vi "未命名 1.vi"() -> ()   [LabVIEW 2013]
panel:
  out "error out":errorcluster
  out "区域最大位移1(mm)":dbl format="%#.1f"
  out "区域最小位移1(mm)":dbl format="%#.1f"
  out "区域最大压力1(KN)":dbl format="%#.3f"
  out "位移监控点1(mm)":dbl format="%#.1f"
  out "监控点最小压力1(KN)":dbl format="%#.3f"
  out "监控点最大压力1(KN)":dbl format="%#.3f"
  out "最小压入位移1(mm)":dbl format="%#.1f"
  out "最大压入位移1(mm)":dbl format="%#.1f"
  out "区域最小压力1(KN)":dbl format="%#.3f"
  out "区域最小压力2(KN)":dbl format="%#.3f"
  out "最小压入位移2(mm)":dbl format="%#.1f"
  out "最大压入位移2(mm)":dbl format="%#.1f"
  out "区域最大压力2(KN)":dbl format="%#.3f"
  out "位移监控点2(mm)":dbl format="%#.1f"
  out "监控点最大压力2(KN)":dbl format="%#.3f"
  out "监控点最小压力2(KN)":dbl format="%#.3f"
  out "区域最小位移2(mm)":dbl format="%#.1f"
  out "区域最大位移2(mm)":dbl format="%#.1f"
  out "伺服1位置设置":dbl format="%#.1f"
  out "伺服2位置设置":dbl format="%#.1f"
  out "吹气时间设置":dbl
  out "喷油时间设置":dbl
  out "伺服2速度设置":dbl format="%#.1f"
  out "伺服1速度设置":dbl format="%#.1f"
  in  "参数加载":bool
  out "ADODB._Connection Out":refnum<k7>
  in  "位移2零点偏移值":dbl format="%#.3f"
  in  "位移2比例偏移值":dbl format="%#.3f"
  in  "压力2比例偏移值":dbl format="%#.3f"
  in  "压力2零点偏移值":dbl format="%#.3f"
  in  "位移1零点偏移值":dbl format="%#.3f"
  in  "位移1比例偏移值":dbl format="%#.3f"
  in  "压力1比例偏移值":dbl format="%#.3f"
  in  "压力1零点偏移值":dbl format="%#.3f"
  in  "停止":bool
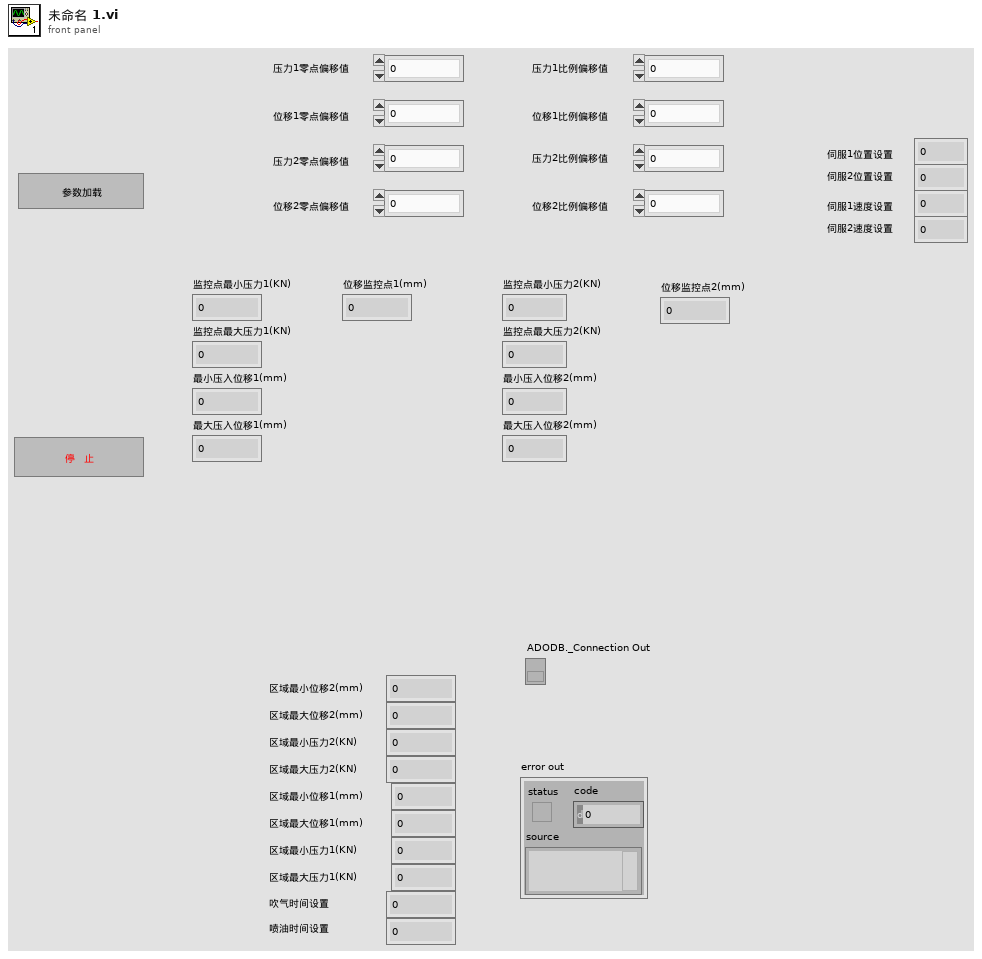
[diagram p1: front panel]
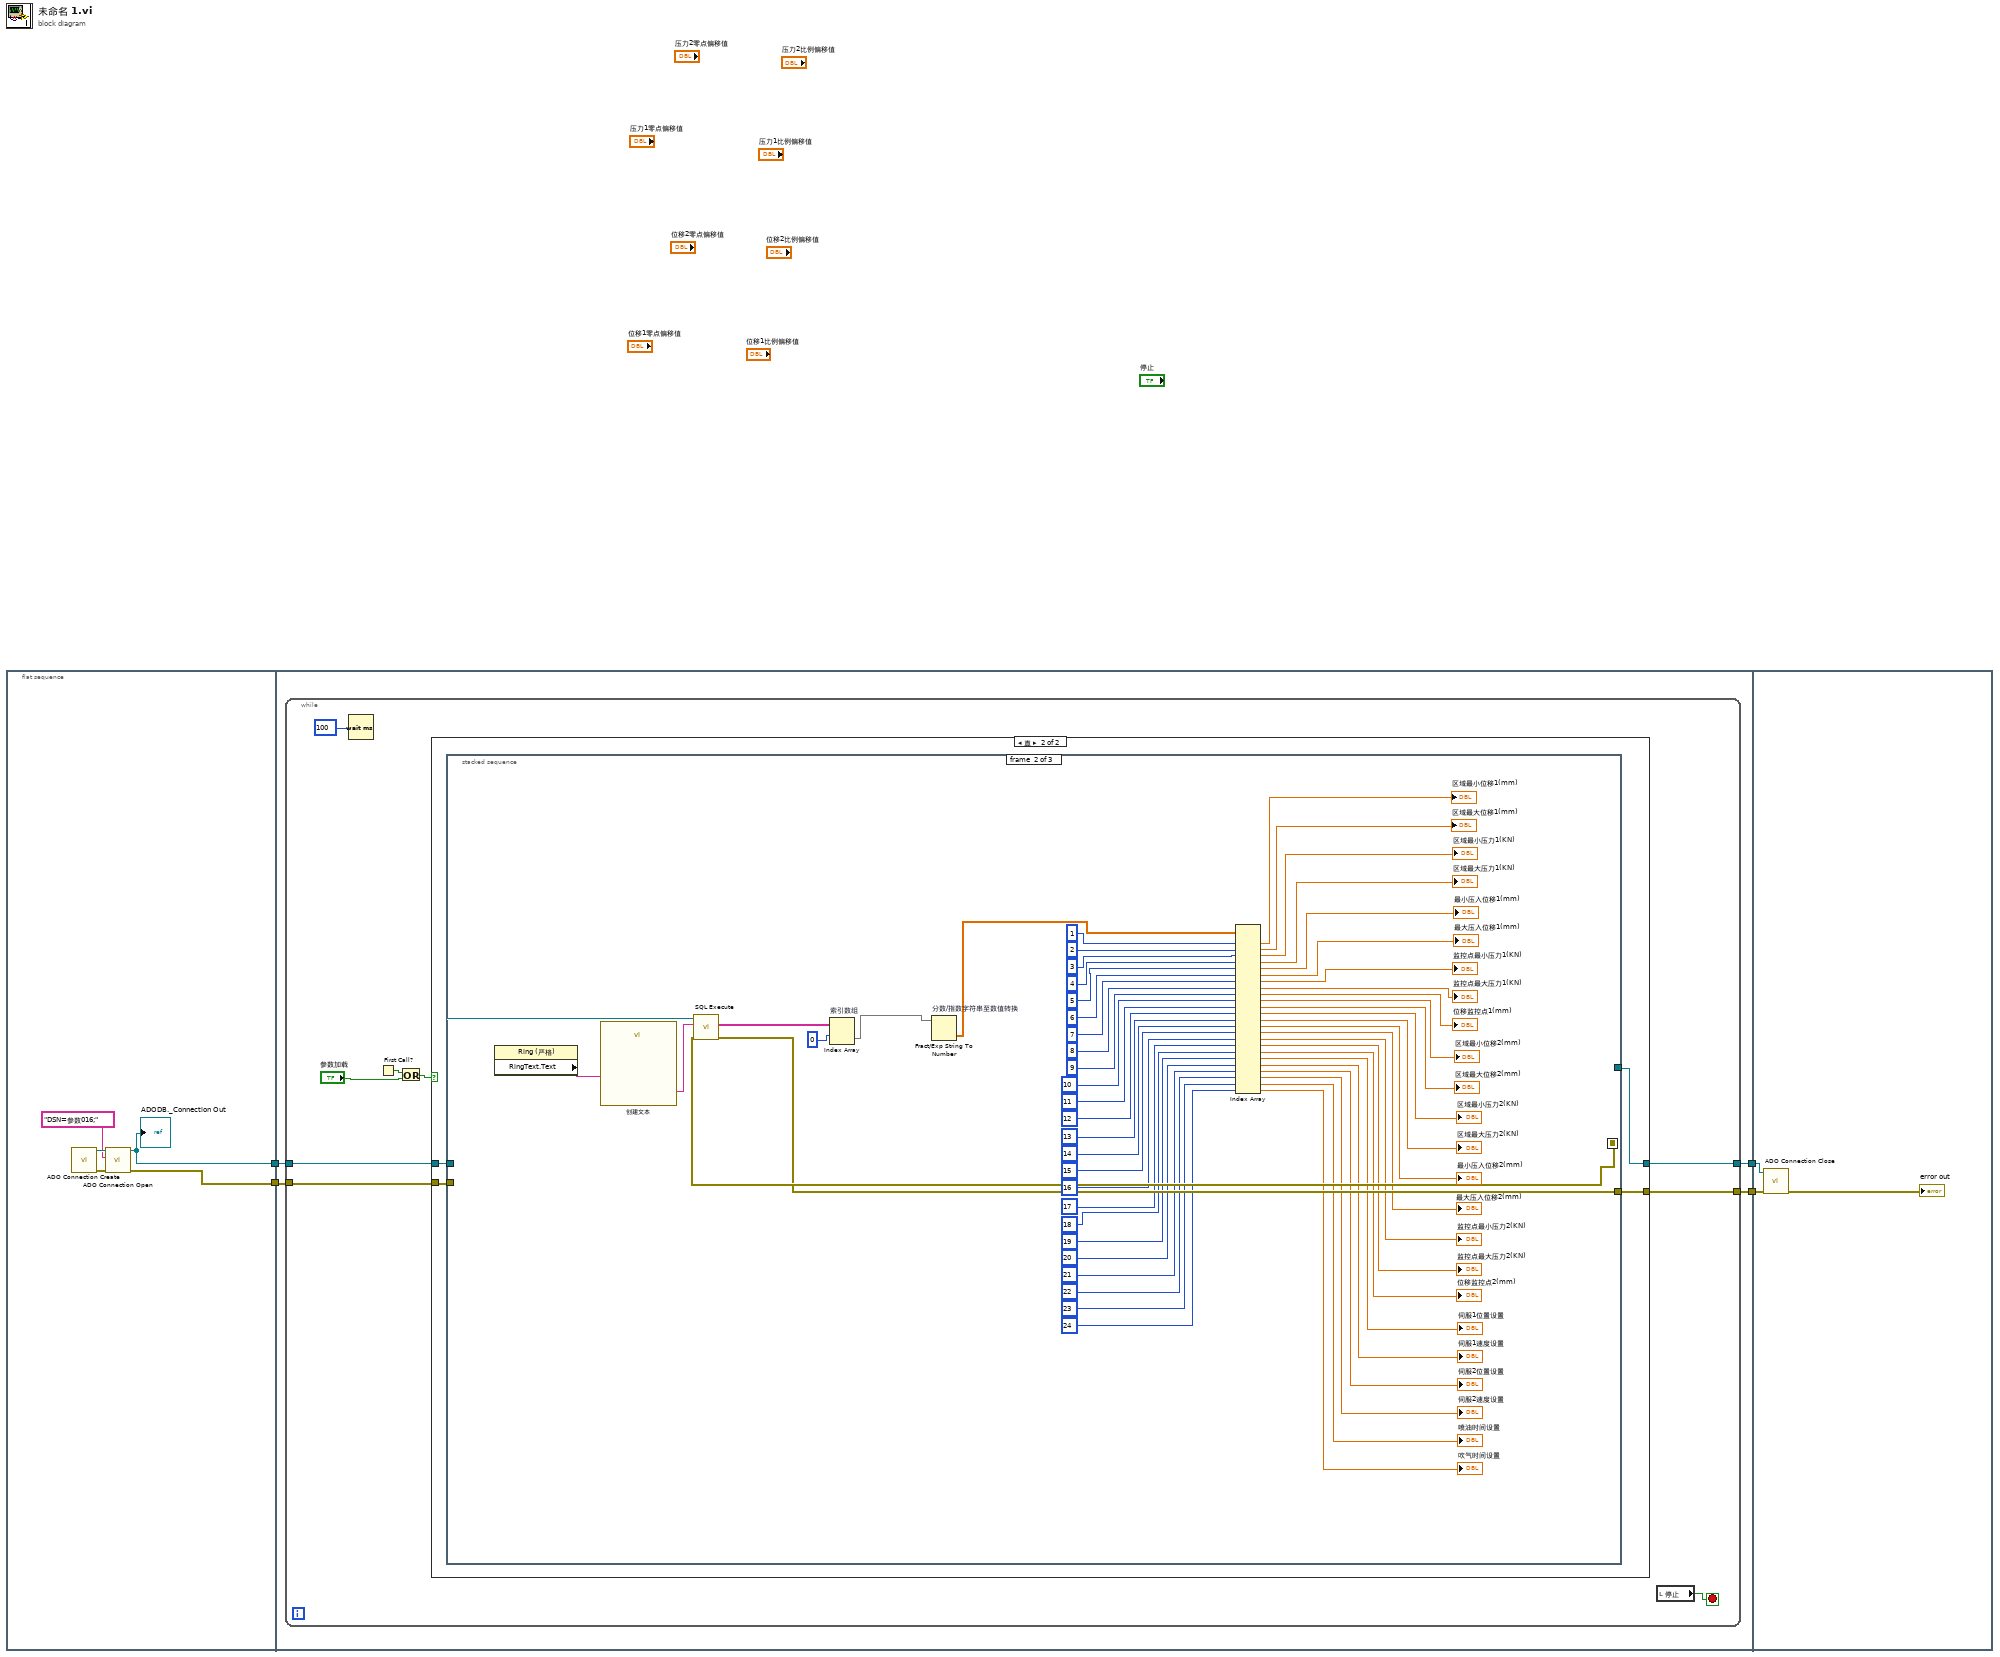
[diagram p0: block diagram]
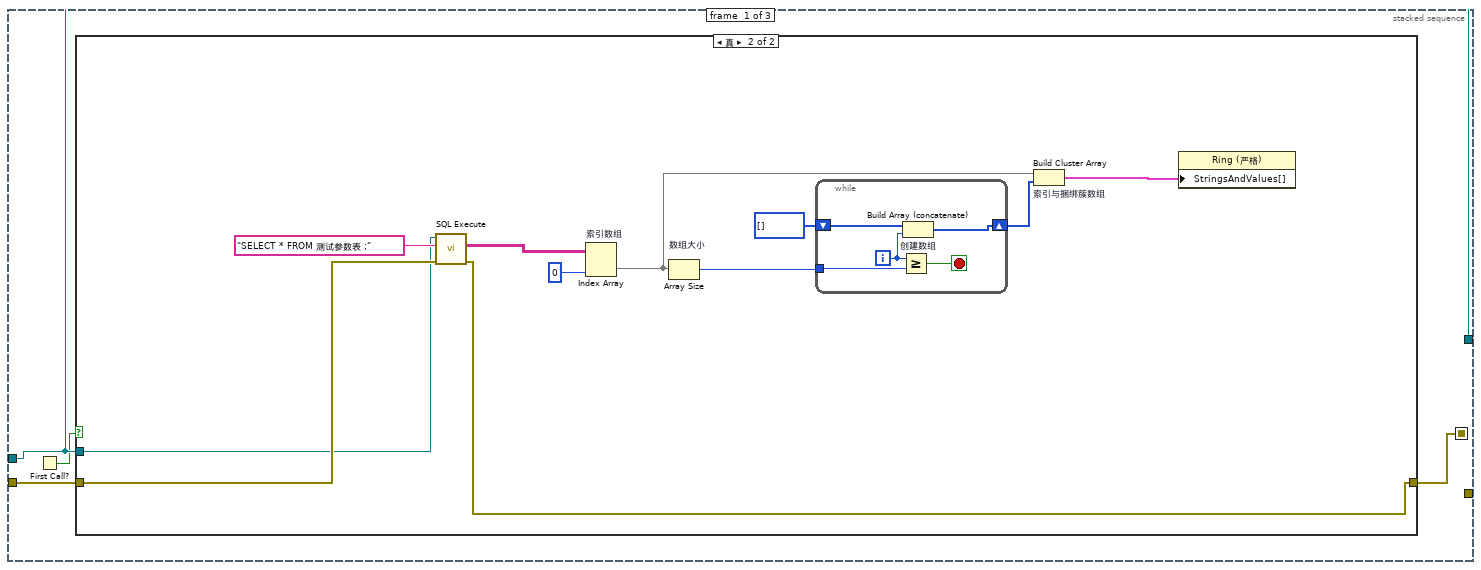
[diagram p3: hidden frame]
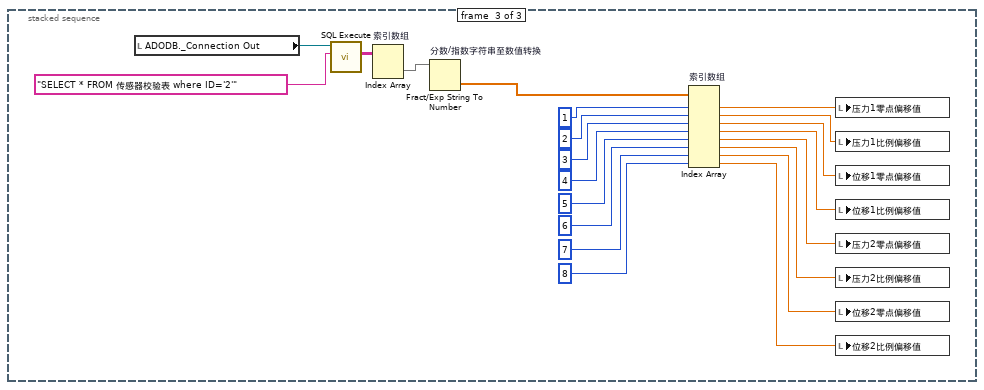
[diagram p5: hidden frame]
diagram:
  n1 = flat-sequence {
    tunnel: [w6] -> w4
    tunnel: [w5] -> w3
    tunnel: w4 -> [w13]
    tunnel: w3 -> [w12]
    tunnel: [w11] -> w2
    tunnel: [w10] -> w1
    tunnel: w2 -> [w129]
    tunnel: w1 -> [w128]
    frame #0 {
      n2 = call "ADO Connection Create.vi"() -> ("error out"=w8:errorcluster, "ADODB._Connection Out"=w9:refnum<k7>)  [unwired: 10 in]
      n3 = call "ADO Connection Open.vi"("error in (no error)"=w8, "ConnectionString"="DSN=参数016;", "ADODB._Connection In"=w9) -> ("error out"=w5:errorcluster, "ADODB._Connection Out"=w6:refnum<k7>)  [unwired: 7 in]
      "ADODB._Connection Out" <- w6
    }
    frame #1 {
      n4 = while {
        tunnel: w13 -> [w18]
        tunnel: w12 -> [w17]
        tunnel: [w16] -> w11
        tunnel: [w15] -> w10
        stop <- w21 stop-if-true
        n5 = Wait (ms)(milliseconds to wait=u32 100 ("等待时间（毫秒）")) -> ()  [unwired: 1 out]
        n6 = First Call?() -> (First Call?: T/F=w20:bool)
        n7 = Or(x=w20, y="参数加载") -> (x .or. y?=w19:bool)
        n8 = case shown="真" w19 {
          tunnel: w18 -> [w24 w28]
          tunnel: w17 -> [w23 w27]
          tunnel: [w24 w26] -> w16
          tunnel: [w23 w25] -> w15
          frame False {
          }
          frame True {
            n9 = stacked-sequence {
              seq-local: [w29 _ _] -> [_ w104 _]
              tunnel: w28 -> [w31 w101 _]
              tunnel: w27 -> [w32 _ _]
              tunnel: [w31 _ _] -> w26
              tunnel: [_ w103 _] -> w25
              frame #0 {
                n10 = First Call?() -> (First Call?: T/F=w30:bool)
                n11 = case shown="真" w30 {
                  tunnel: w32 -> [w33 w38]
                  tunnel: w31 -> [_ w36]
                  tunnel: [w33 w35] -> w29
                  frame False {
                  }
                  frame True {
                    n12 = call "SQL Execute.vi"("error in (no error)"=w38, "Command Text"="SELECT * FROM 测试参数表 ;", "ADODB._Connection In"=w36) -> ("error out"=w35:errorcluster, "Data"=w39:string[][])  [unwired: 5 in, 2 out]
                    n13 = Index Array "索引数组"(array=w39, index (col)=0 ("禁用的索引 (列)")) -> (element=w42:string[])  [unwired: 1 in]
                    n14 = Array Size "数组大小"(array=w42) -> (size(s)=w41:i32)
                    n15 = while {
                      shift-right: [w47] -> w40
                      shift-left: i32[] [] -> [w48]
                      tunnel: w41 -> [w45]
                      i -> [w46]
                      stop <- w49 stop-if-true
                      n16 = Greater Or Equal?(x=w46, y=w45) -> (x >= y?=w49:bool)
                      n17 = Build Array (concatenate) "创建数组"(w48, w46) -> (w47:i32[])
                    }
                    n18 = Build Cluster Array "索引与捆绑簇数组"(w42, w40) -> (w34:cluster{"String":string, i32}[])
                    n19 = property on="属性节点" class="Ring (严格)"("StringsAndValues[]"=w34) -> ()  [unwired: 2 in, 2 out]
                  }
                }
              }
              frame #1 {
                n20 = property on="属性节点" class="Ring (严格)"() -> ("RingText.Text"=w100:string)  [unwired: 2 in, 2 out]
                n21 = call "创建文本"("产品型号"=w100) -> ("Result"=w102:string)  [unwired: 13 in, 1 out]
                n22 = call "SQL Execute.vi"("error in (no error)"=w104, "Command Text"=w102, "ADODB._Connection In"=w101) -> ("error out"=w103:errorcluster, "Data"=w106:string[][])  [unwired: 5 in, 2 out]
                n23 = Index Array "索引数组"(array=w106, index (row)=0 ("索引 (行)")) -> (element=w99:string[])  [unwired: 1 in]
                n24 = Fract/Exp String To Number "分数/指数字符串至数值转换"(string=w99) -> (number=w50:dbl[])  [unwired: 3 in, 1 out]
                n25 = Index Array(array=w50, index #1=1 ("索引"), index #2=2 ("索引"), index #3=3 ("索引"), index #4=4 ("索引"), index #5=5 ("索引"), index #6=6 ("索引"), index #7=7 ("索引"), index #8=8 ("索引"), index #9=9 ("索引"), index #10=10 ("索引"), index #11=11 ("索引"), index #12=12 ("索引"), index #13=13 ("索引"), index #14=14 ("索引"), index #15=15 ("索引"), index #16=16 ("索引"), index #17=17 ("索引"), index #18=18 ("索引"), index #19=19 ("索引"), index #20=20 ("索引"), index #21=21 ("索引"), index #22=22 ("索引"), index #23=23 ("索引"), index #24=24 ("索引")) -> (element #1=→"区域最小位移1(mm)":dbl, element #2=→"区域最大位移1(mm)":dbl, element #3=→"区域最小压力1(KN)":dbl, element #4=→"区域最大压力1(KN)":dbl, element #5=→"最小压入位移1(mm)":dbl, element #6=→"最大压入位移1(mm)":dbl, element #7=→"监控点最小压力1(KN)":dbl, element #8=→"监控点最大压力1(KN)":dbl, element #9=→"位移监控点1(mm)":dbl, element #10=→"区域最小位移2(mm)":dbl, element #11=→"区域最大位移2(mm)":dbl, element #12=→"区域最小压力2(KN)":dbl, element #13=→"区域最大压力2(KN)":dbl, element #14=→"最小压入位移2(mm)":dbl, element #15=→"最大压入位移2(mm)":dbl, element #16=→"监控点最小压力2(KN)":dbl, element #17=→"监控点最大压力2(KN)":dbl, element #18=→"位移监控点2(mm)":dbl, element #19=→"伺服1位置设置":dbl, element #20=→"伺服1速度设置":dbl, element #21=→"伺服2位置设置":dbl, element #22=→"伺服2速度设置":dbl, element #23=→"喷油时间设置":dbl, element #24=→"吹气时间设置":dbl)
              }
              frame #2 {
                n26 = local read "ADODB._Connection Out"() -> (w122:refnum<k7>)
                n27 = call "SQL Execute.vi"("Command Text"="SELECT * FROM 传感器校验表 where ID='2'", "ADODB._Connection In"=w122) -> ("Data"=w127:string[][])  [unwired: 6 in, 3 out]
                n28 = Index Array "索引数组"(array=w127) -> (element=w126:string[])  [unwired: 2 in]
                n29 = Fract/Exp String To Number "分数/指数字符串至数值转换"(string=w126) -> (number=w125:dbl[])  [unwired: 3 in, 1 out]
                n30 = Index Array "索引数组"(array=w125, index #1=1 ("索引"), index #2=2 ("索引"), index #3=3 ("索引"), index #4=4 ("索引"), index #5=5 ("索引"), index #6=6 ("索引"), index #7=7 ("索引"), index #8=8 ("索引")) -> (element #1=w114:dbl, element #2=w113:dbl, element #3=w112:dbl, element #4=w111:dbl, element #5=w110:dbl, element #6=w109:dbl, element #7=w108:dbl, element #8=w107:dbl)
                n31 = local write "压力1零点偏移值"(w114) -> ()
                n32 = local write "压力1比例偏移值"(w113) -> ()
                n33 = local write "位移1零点偏移值"(w112) -> ()
                n34 = local write "位移1比例偏移值"(w111) -> ()
                n35 = local write "压力2零点偏移值"(w110) -> ()
                n36 = local write "压力2比例偏移值"(w109) -> ()
                n37 = local write "位移2零点偏移值"(w108) -> ()
                n38 = local write "位移2比例偏移值"(w107) -> ()
              }
            }
          }
        }
        n39 = local read "停止"() -> (w21:bool)
      }
    }
    frame #2 {
      n40 = call "ADO Connection Close.vi"("error in (no error)"=w128, "ADODB._Connection In"=w129) -> ("error out"=→"error out":errorcluster)  [unwired: 8 in, 1 out]
    }
  }
